vi "manual test UI.vi"(8 "error in (no error)":errorcluster caption="Fehler (Eingang, kein Fehler)", 11 "TestInterface Eingang":refnum<class "TestInterface.lvclass"> caption="DNL_LabVIEW Object in") -> (0 "error out":errorcluster caption="Fehler (Ausgang)", 1 "parameters":string[][](table), 2 "Parameters":u32[](array[numeric]), 3 "TestInterface Ausgang":refnum<class "TestInterface.lvclass"> caption="DNL_LabVIEW Object out", 5 "abbrechen":bool)   [LabVIEW 2013, in "TestInterface.lvclass"]
uses:
  TestInterface.lvclass
  HF-Felder/modulation.ctl
  HF-Felder/HF-Felder.lvclass
panel:
  in  "parameters 2":string[][](table)
  in  "ok":bool
  in  "abbrechen":bool
  in  "Enum":T1
  # "Dies ist lediglich eine Vorlage..."
  # "Auswahlmenü"
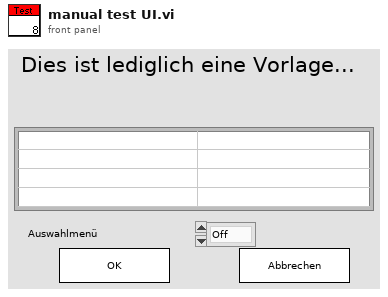
[diagram p1: front panel]
types:
  T1 = typedef "HF-Felder.lvclass/modulation.ctl" = enum16{"Off", "2Hz", "400Hz", "1kHz", "Pulse"}
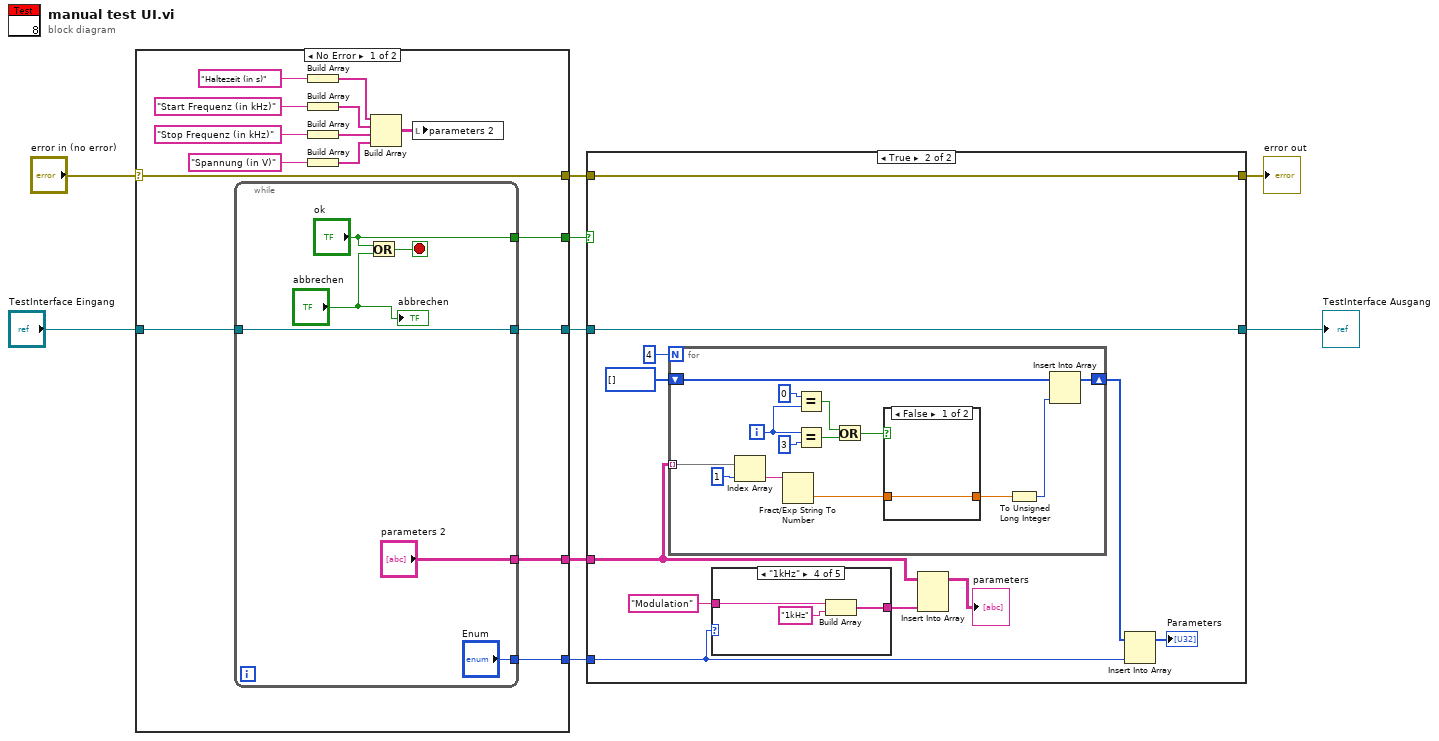
[diagram p0: block diagram]
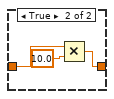
[diagram p3: hidden frame]
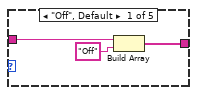
[diagram p4: hidden frame]
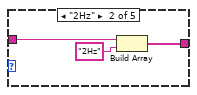
[diagram p5: hidden frame]
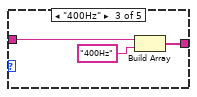
[diagram p6: hidden frame]
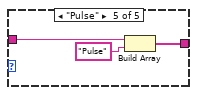
[diagram p7: hidden frame]
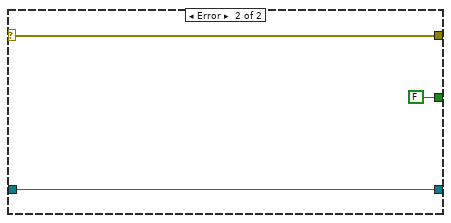
[diagram p8: hidden frame]
diagram:
  n1 = case shown="No Error" "error in (no error)" {
    selector: "error in (no error)" -> [w22 w33]
    tunnel: [w24 w32] -> w6
    tunnel: "TestInterface Eingang" -> [w23 w32]
    tunnel: [w22 w33] -> w5
    tunnel: [w21 _] -> w8
    tunnel: [w20 _] -> w9
    tunnel: [w19 FALSE ("ok")] -> w7
    frame No Error {
      n2 = while {
        tunnel: [w29] -> w24
        tunnel: w23 -> [w29]
        tunnel: ["parameters 2"] -> w21
        tunnel: ["Enum"] -> w20
        tunnel: ["ok"] -> w19
        stop <- w30 stop-if-true
        n3 = Or(x="ok", y="abbrechen") -> (x .or. y?=w30:bool)
        "abbrechen" <- "abbrechen"
      }
      n4 = Build Array("Haltezeit (in s)") -> (w17:string[])
      n5 = Build Array("Start Frequenz (in kHz)") -> (w10:string[])
      n6 = Build Array("Stop Frequenz (in kHz)") -> (w11:string[])
      n7 = Build Array("Spannung (in V)") -> (w12:string[])
      n8 = Build Array(w17, w10, w11, w12) -> (w16:string[][])
      n9 = local write "parameters 2"(w16) -> ()
    }
    frame Error {
    }
  }
  n10 = case shown="True" w7 {
    tunnel: w9 -> [_ w41]
    tunnel: w8 -> [_ w43]
    tunnel: w6 -> [w35 w36]
    tunnel: [w35 w36] -> w2
    tunnel: w5 -> [w34 w37]
    tunnel: [w34 w37] -> w1
    frame False {
    }
    frame True {
      n11 = for {
        N: 4 -> [_]
        tunnel: w43 -> [w60] mode=indexing
        shift-right: [w50] -> w40
        shift-left: u32[] [] -> [w51]
        i -> [w47]
        n12 = Index Array(array=w60, index=1 ("Index")) -> (element=w58:string)
        n13 = Fract/Exp String To Number(string=w58) -> (number=w52:dbl)  [unwired: 3 in, 1 out]
        n14 = Equal?(x=u32 0, y=w47) -> (x = y?=w57:bool)
        n15 = Equal?(x=w47, y=u32 3) -> (x = y?=w56:bool)
        n16 = Or(x=w57, y=w56) -> (x .or. y?=w53:bool)
        n17 = case shown="False" w53 {
          tunnel: w52 -> [w61 w64]
          tunnel: [w61 w62] -> w49
          frame False {
          }
          frame True {
            n18 = Multiply(x=w64, y=10.0) -> (x*y=w62:dbl)
          }
        }
        n19 = To Unsigned Long Integer(number=w49) -> (unsigned 32bit integer=w48:u32)
        n20 = Insert Into Array(array=w51, new element=w48) -> (w50:u32[])  [unwired: 1 in]
      }
      n21 = case shown="\"1kHz\"" w41 {
        tunnel: "Modulation" -> [w67 w69 w72 w75 w78]
        tunnel: [w65 w68 w71 w74 w77] -> w45
        frame "Off", Default {
          n22 = Build Array(w67, "Off" ("Element")) -> (w65:string[])
        }
        frame "2Hz" {
          n23 = Build Array(w69, "2Hz" ("Element")) -> (w68:string[])
        }
        frame "400Hz" {
          n24 = Build Array(w72, "400Hz" ("Element")) -> (w71:string[])
        }
        frame "1kHz" {
          n25 = Build Array(w75, "1kHz" ("Element")) -> (w74:string[])
        }
        frame "Pulse" {
          n26 = Build Array(w78, "Pulse" ("Element")) -> (w77:string[])
        }
      }
      n27 = Insert Into Array(array=w43, new element=w45) -> (→"parameters":string[][])  [unwired: 2 in]
      n28 = Insert Into Array(array=w40, new element=w41) -> (→"Parameters":u32[])  [unwired: 1 in]
    }
  }
  "error out" <- w1
  "TestInterface Ausgang" <- w2
